vi "Ensure All Modules Exit.vi"(8 "Error in":errorcluster caption="Error in (no error)") -> (0 "Error out":errorcluster)   [LabVIEW 2017]
uses:
  src/user.lib/_NEVSTOP/Communicable State Machine(CSM)/_Support/Typedef/_CSM_List Module Scope.ctl
  src/user.lib/_NEVSTOP/Communicable State Machine(CSM)/Communicable State Machine.lvlib
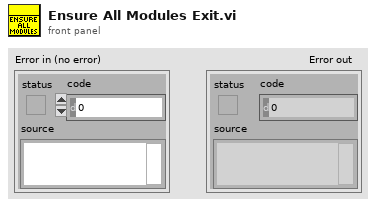
[diagram p1: front panel]
types:
  T1 = typedef "Communicable State Machine.lvlib/_CSM_List Module Scope.ctl" = enum16{"Normal", "System Only", "All"}
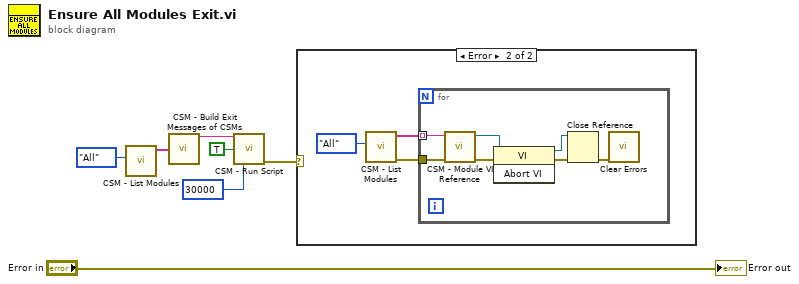
[diagram p0: block diagram]
diagram:
  n1 = call "CSM - List Modules.vi"("Scope (Normal)"=_CSM_List_Module_Scope."All") -> ("Module Names"=w4:string[])  [unwired: 9 in, 1 out]
  n2 = call "CSM - Build Exit Messages of CSMs.vi"("CSMs"=w4) -> ("States"=w6:string)  [unwired: 14 in]
  n3 = call "CSM - Run Script.vi"("CSM Scripts"=w6, "Continue If Error? (F)"=TRUE ("Continue If Error?(F)"), "Response Timeout (-2 Using Global Settings)"=30000) -> ("error out"=w2:errorcluster)  [unwired: 10 in, 2 out]
  n4 = case shown="Error" w2 {
    frame No Error {
    }
    frame Error {
      n5 = call "CSM - List Modules.vi"("Scope (Normal)"=_CSM_List_Module_Scope."All") -> ("error out"=w9:errorcluster, "Module Names"=w8:string[])  [unwired: 9 in]
      n6 = for {
        tunnel: w9 -> [w17]
        tunnel: w8 -> [w16] mode=indexing
        n7 = call "CSM - Module VI Reference.vi"("error in (no error)"=w17, "CSM Name"=w16) -> ("error out"=w14:errorcluster, "CSM Module VIRef"=w15:refnum<vi>)  [unwired: 8 in]
        n8 = invoke class="VI" method="Abort VI"(reference=w15, error in=w14) -> (reference out=w12:refnum<vi>, error out=w13:errorcluster)  [unwired: 1 in, 1 out]
        n9 = Close Reference(reference=w12, error in (no error)=w13) -> (error out=w11:errorcluster)
        n10 = call <vilib>:"Clear Errors.vi"("error in (no error)"=w11) -> ()  [unwired: 5 in, 2 out]
      }
    }
  }
  "Error out" <- "Error in"
